vi "S8300E_COMPARE_LANMAC_SFCS_Auto.vi"() -> ()   [LabVIEW 2011]
panel:
  out "Expected MAC":string[](array[string])
  out "PORT1_MAC":string
  out "UUT MAC List":string
  out "CMD-LIST":cluster{string, string, string, string}[](array[cluster])
  out "log msg":string
  out "VISA resource name out":refnum<visa-resource-name>
  out "BEGIN TIME":u32
  out "進行狀況":string
  # "Error Code:MAC-PORT1\nError Code:MAC-PORT2\nError Code:MAC-PORT3"
  # "2014-12-12"
  # "S8300E UUT 3 Ports MAC (接UART COM9)"
  # "Step1:PQAW_MAC.LOG  contains MAC1 information\nStep2:Compare UUT MAC with PQAW_MAC.Log"
  # "Auto-Test\n自動測試"
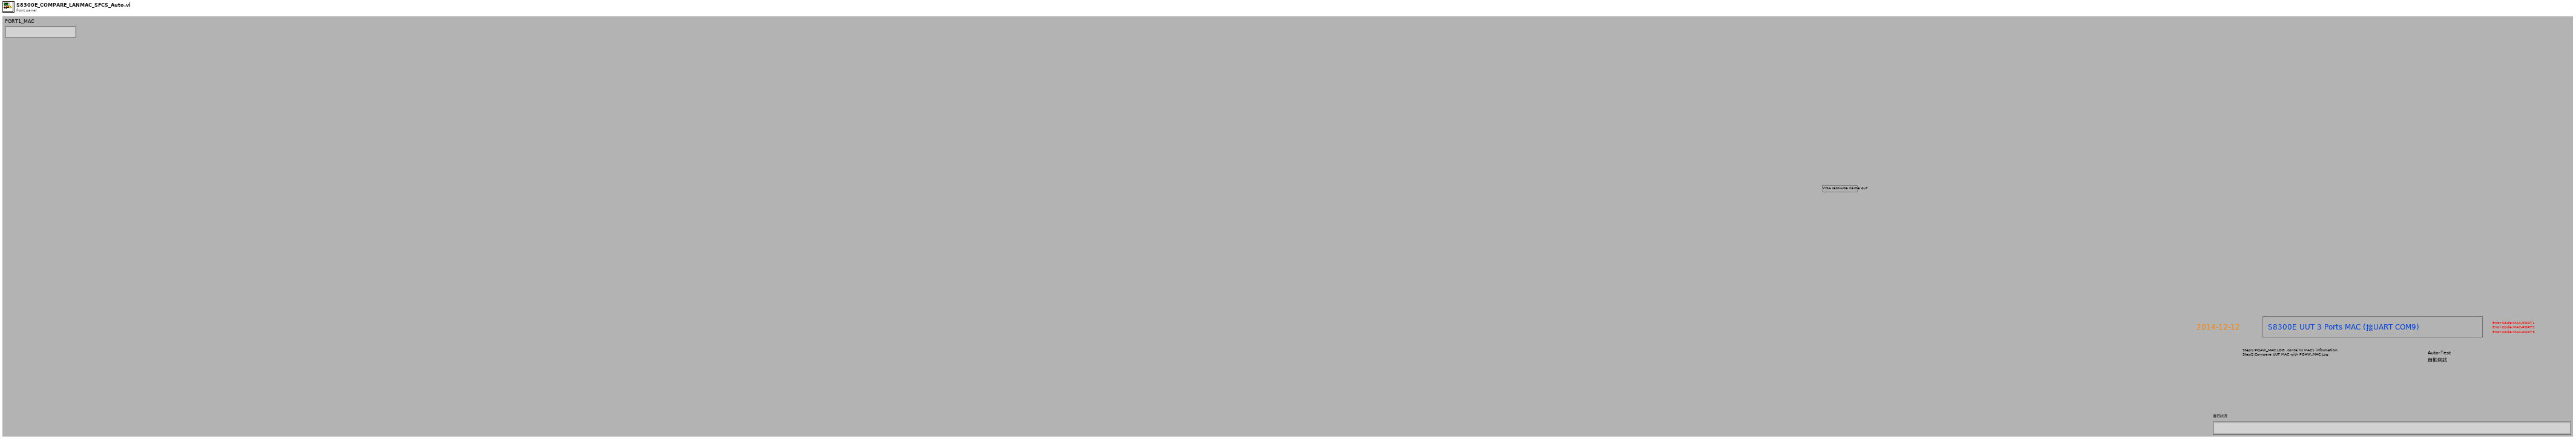
[diagram p1: front panel]
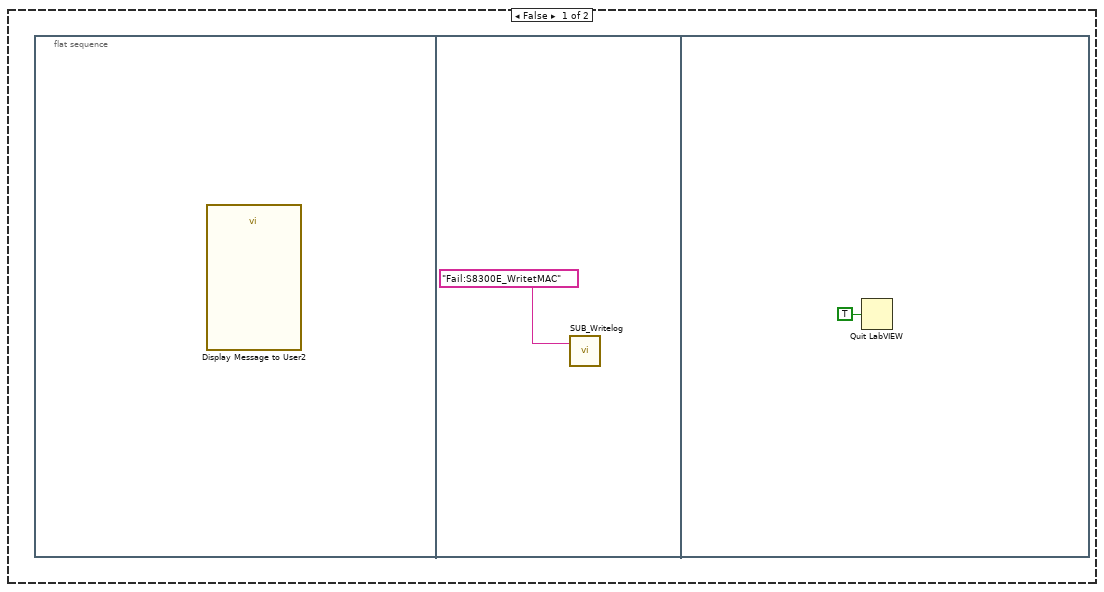
[diagram p3: hidden frame]
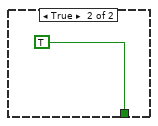
[diagram p9: hidden frame]
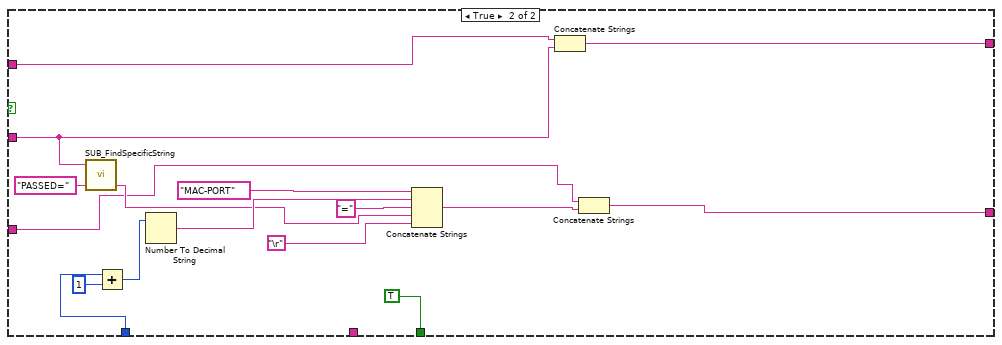
[diagram p11: hidden frame]
diagram:
  n1 = flat-sequence {
    frame #0 {
      n2 = Tick Count (ms)() -> (millisecond timer value=→"BEGIN TIME":u32)
    }
    frame #1 {
      n3 = property on="進行狀況" class="Str"("Blinking"=TRUE) -> ()  [unwired: 2 in, 2 out]
      "進行狀況" <- "進入測試準備中...." ("進行狀況")
      "PORT1_MAC" <- ""
    }
    frame #2 {
      n4 = call "SUB_SearchFile_inFolder.vi"("Search Filename in Folder"="S8300E_sfcs_misc.txt") -> ("File Existing True/Flase"=w5:bool)  [unwired: 1 in]
      n5 = case shown="False" w5 {
        frame False {
          n6 = flat-sequence {
            frame #0 {
              n7 = call "Display Message to User"() -> ()  [unwired: 10 in, 2 out]
            }
            frame #1 {
              n8 = call "SUB_Writelog.vi"("Pass/Fail"="Fail:S8300E_COMPARE_LANMAC_SFCS_Auto") -> ()  [unwired: 2 in]
            }
            frame #2 {
              n9 = Quit LabVIEW(quit? (T)=TRUE) -> ()
            }
          }
        }
        frame True {
        }
      }
    }
    frame #3 {
      n10 = call "SUB_SearchFile_inFolder.vi"("Search Filename in Folder"="PQAW_MAC.LOG") -> ("File Existing True/Flase"=w9:bool)  [unwired: 1 in]
      n11 = case shown="True" w9 {
        frame False {
          n12 = flat-sequence {
            frame #0 {
              n13 = call "Display Message to User2"() -> ()  [unwired: 10 in, 2 out]
            }
            frame #1 {
              n14 = call "SUB_Writelog.vi"("Pass/Fail"="Fail:S8300E_WritetMAC") -> ()  [unwired: 2 in]
            }
            frame #2 {
              n15 = Quit LabVIEW(quit? (T)=TRUE) -> ()
            }
          }
        }
        frame True {
          n16 = call "SUB_Read_specifFile.vi"("name or relative path"="PQAW_MAC.LOG" ("Search Filename in Folder")) -> ("text"=w20:string)  [unwired: 1 in, 1 out]
          n17 = call "SUB_FindSpecificString.vi"("Find this String"="LAN_MAC=", "String data"=w20) -> ("before \"; \" string"=w18:string, "Found"=w14:bool)  [unwired: 2 in]
          n18 = local write "PORT1_MAC"(w18) -> ()
          n19 = String Length(string=w18) -> (length=w17:i32)
          n20 = Equal?(x=w17, y=12) -> (x = y?=w13:bool)
          n21 = And(x=w14, y=w13) -> (x .and. y?=w15:bool)
          n22 = case shown="False" w15 {
            frame False {
              n23 = flat-sequence {
                frame #0 {
                  n24 = call "Display Message to User3"() -> ()  [unwired: 10 in, 2 out]
                }
                frame #1 {
                  n25 = call "SUB_Writelog.vi"("Pass/Fail"="Fail:S8300E_COMPARE_LANMAC_SFCS_Auto") -> ()  [unwired: 2 in]
                }
                frame #2 {
                  n26 = Quit LabVIEW(quit? (T)=TRUE) -> ()
                }
              }
            }
            frame True {
            }
          }
        }
      }
    }
    frame #4 {
      n27 = local read "PORT1_MAC"() -> (w34:string)
      n28 = call "SUB_Gen3ports_MACString.vi"("Port1-MAC Input"=w34) -> ("port3-MAC"=w25:string, "port2-MAC"=w26:string, "port1-MAC"=w27:string)  [unwired: 2 in]
      n29 = Concatenate Strings("./mac.sh -r -e  1", "\r") -> (w51:string)
      n30 = Concatenate Strings("PASSED=", w27) -> (w32:string)
      n31 = Concatenate Strings("PASSED=", w26) -> (w30:string)
      n32 = Concatenate Strings("./mac.sh -r -e  2", "\r") -> (w47:string)
      n33 = Concatenate Strings("PASSED=", w25) -> (w28:string)
      n34 = Concatenate Strings("./mac.sh -r -e  3", "\r") -> (w43:string)
      n35 = Bundle(w51, w32, "Checking MAC-PORT1..", "MAC-PORT1") -> (w38:cluster{string, string, string, string})  [unwired: 1 in]
      n36 = Bundle(w47, w30, "Checking MAC-PORT2...", "MAC-PORT2") -> (w37:cluster{string, string, string, string})  [unwired: 1 in]
      n37 = Build Array(w27, w26, w25) -> (→"Expected MAC":string[])
      n38 = Bundle(w43, w28, "Checking MAC-PORT3...", "MAC-PORT3") -> (w36:cluster{string, string, string, string})  [unwired: 1 in]
      n39 = Build Array(w38, w37, w36) -> (→"CMD-LIST":cluster{string, string, string, string}[])
    }
    frame #5 {
      n40 = case shown="True" TRUE {
        frame False {
        }
        frame True {
          n41 = call "SUB_COM1_CLOSE.vi"("VISA resource name"=refnum<visa-resource-name> "COM9") -> ()  [unwired: 3 in]
        }
      }
    }
    frame #6 {
      n42 = case shown="True" TRUE {
        frame False {
        }
        frame True {
          w58 = "\r"
          n43 = call "SUB_COM9_INIT.vi"("baud rate"=u32 115200) -> ("VISA resource name out"=w62:refnum<visa-resource-name>)  [unwired: 1 in, 1 out]
          "VISA resource name out" <- w62
          n44 = Concatenate Strings(w58, w58, w58) -> (w57:string)
          n45 = call "SUB_COM1Wrt.vi"("VISA resource name"=w62, "write buffer"=w57) -> ("duplicate VISA resource name"=w59:refnum<visa-resource-name>)  [unwired: 1 in, 1 out]
          n46 = call "SUB_ContinueCom1Read.vi"("Numeric"=1200, "duplicate VISA resource name 2"=w59) -> ()  [unwired: 1 in, 3 out]
        }
      }
    }
    frame #7 {
      n47 = case shown="True" TRUE {
        frame False {
        }
        frame True {
          n48 = while {
            stop <- w73 stop-if-true
            w64 = "\r"
            n49 = local read "VISA resource name out"() -> (w66:refnum<visa-resource-name>)
            n50 = Tick Count (ms)() -> (millisecond timer value=w71:u32)
            n51 = Concatenate Strings(w64, w64, w64) -> (w65:string)
            n52 = call "SUB_COM1Wrt.vi"("VISA resource name"=w66, "write buffer"=w65) -> ("duplicate VISA resource name"=w72:refnum<visa-resource-name>)  [unwired: 1 in, 1 out]
            n53 = call "SUB_READ_COM1_FindString_timeout.vi"("Find this String"="s8300e_func_test#", "Timeout Seccond"=2.0, "Begin time"=w71, "duplicate VISA resource name 2"=w72) -> ("Output String"=w67:string, "Found String"=w68:bool)  [unwired: 1 in, 1 out]
            n54 = case shown="False" w68 {
              tunnel: [w75 TRUE] -> w73
              tunnel: w67 -> [w74 _]
              frame False {
                n55 = call "SUB_YESNO.vi"("Debug View"=w74, "Status"="UART無正確反應!需有S8300E字串") -> ("yes/no"=w78:enum32{"No Selection", "Yes", "No", "None"})  [unwired: 1 in]
                n56 = Equal?(x=w78, y=enum32{"No Selection", "Yes", "No", "None"}."No") -> (x = y?=w76:bool)
                n57 = case shown="True" w76 {
                  tunnel: [_ w80] -> w75
                  frame False {
                  }
                  frame True {
                    n58 = flat-sequence {
                      tunnel: [w84] -> w80
                      frame #0 {
                        n59 = call "SUB_Writelog.vi"("Pass/Fail"="Fail:S8300E_COMPARE_LANMAC_SFCS_Auto") -> ()  [unwired: 2 in]
                      }
                      frame #1 {
                        n60 = call "SUB_SFCS_SendResult.vi"("ErrorCode"="UART", "PASS_Fail (1/0)"=i8 0) -> ()  [unwired: 1 out]
                      }
                      frame #2 {
                        w84 = TRUE ("quit? (T)")
                        n61 = Quit LabVIEW(quit? (T)=w84) -> ()
                      }
                    }
                  }
                }
              }
              frame True {
              }
            }
          }
        }
      }
    }
    frame #8 {
      n62 = local read "CMD-LIST"() -> (w88:cluster{string, string, string, string}[])
      n63 = Array Size(array=w88) -> (size(s)=w91:i32)
      n64 = for {
        N: w91 -> [_]
        shift-right: [w96] -> w89
        shift-left: "" -> [w95]
        shift-right: [w93] -> w86
        shift-left: "" -> [w92]
        i -> [w94]
        n65 = while {
          tunnel: w94 -> [w115]
          tunnel: [w107] -> w96
          tunnel: w95 -> [w106]
          tunnel: w94 -> [w99]
          tunnel: [w98] -> w93
          tunnel: w92 -> [w97]
          stop <- w109 stop-if-true
          n66 = local read "VISA resource name out"() -> (w111:refnum<visa-resource-name>)
          n67 = local read "CMD-LIST"() -> (w105:cluster{string, string, string, string}[])
          n68 = Index Array(array=w105, index=w115) -> (element=w104:cluster{string, string, string, string})
          n69 = Unbundle(w104) -> (w103:string, w101:string, w102:string, w100:string)
          n70 = call "SUB_COM1Wrt.vi"("VISA resource name"=w111, "write buffer"=w103) -> ("duplicate VISA resource name"=w114:refnum<visa-resource-name>)  [unwired: 1 in, 1 out]
          n71 = Tick Count (ms)() -> (millisecond timer value=w113:u32)
          n72 = call "SUB_READ_COM1_FindString_timeout.vi"("Find this String"=w101, "Timeout Seccond"=2.0, "Begin time"=w113, "duplicate VISA resource name 2"=w114) -> ("Output String"=w108:string, "Found String"=w110:bool)  [unwired: 1 in, 1 out]
          n73 = local write "進行狀況"(w102) -> ()
          n74 = case shown="False" w110 {
            tunnel: [_ TRUE] -> w109
            tunnel: w108 -> [w117 w151]
            tunnel: [w131 w156] -> w107
            tunnel: w106 -> [w131 w155]
            tunnel: w100 -> [w130 _]
            tunnel: w99 -> [w124 w147]
            tunnel: [w126 w143] -> w98
            tunnel: w97 -> [w126 w142]
            frame False {
              n75 = local read "Expected MAC"() -> (w125:string[])
              n76 = local read "進行狀況"() -> (w128:string)
              n77 = Concatenate Strings("如下系統回傳值" ("string"), "\r", w117) -> (w116:string)
              n78 = Index Array(array=w125, index=w124) -> (element=w122:string)
              n79 = Concatenate Strings("期望MAC 值=" ("string"), w122, "\r") -> (w120:string)
              n80 = Concatenate Strings(w120, "\r", w128) -> (w127:string)
              n81 = call "SUB_YESNO.vi"("Debug View"=w116, "Status"=w127) -> ("yes/no"=w134:enum32{"No Selection", "Yes", "No", "None"})  [unwired: 1 in]
              n82 = Equal?(x=w134, y=enum32{"No Selection", "Yes", "No", "None"}."No") -> (x = y?=w132:bool)
              n83 = case shown="True" w132 {
                tunnel: w130 -> [_ w135]
                frame False {
                }
                frame True {
                  n84 = flat-sequence {
                    tunnel: [w137] -> w136
                    tunnel: w135 -> [w137]
                    tunnel: w136 -> [w139]
                    frame #0 {
                      n85 = call "SUB_Writelog.vi"("Pass/Fail"="Fail:S8300E_COMPARE_LANMAC_SFCS_Auto") -> ()  [unwired: 2 in]
                    }
                    frame #1 {
                      n86 = call "SUB_SFCS_SendResult.vi"("ErrorCode"=w139, "PASS_Fail (1/0)"=i8 0) -> ()  [unwired: 1 out]
                    }
                    frame #2 {
                      n87 = Quit LabVIEW(quit? (T)=TRUE) -> ()
                    }
                  }
                }
              }
            }
            frame True {
              n88 = call "SUB_FindSpecificString.vi"("Find this String"="PASSED=", "String data"=w151) -> ("before \"; \" string"=w149:string)  [unwired: 2 in, 1 out]
              n89 = Add(x=w147, y=1) -> (x+y=w145:i32)
              n90 = Number To Decimal String(number=w145) -> (decimal integer string=w153:string)  [unwired: 1 in]
              n91 = Concatenate Strings("MAC-PORT" ("string"), w153, "=" ("string"), w149, "\r") -> (w144:string)
              n92 = Concatenate Strings(w155, w151) -> (w156:string)
              n93 = Concatenate Strings(w142, w144) -> (w143:string)
            }
          }
        }
      }
      "log msg" <- w89
      "UUT MAC List" <- w86
    }
    frame #9 {
      n94 = call "SUB_COM1_CLOSE.vi"("VISA resource name"=refnum<visa-resource-name> "COM9") -> ()  [unwired: 3 in]
    }
    frame #10 {
      n95 = local read "log msg"() -> (w159:string)
      n96 = local read "BEGIN TIME"() -> (w165:u32)
      n97 = Tick Count (ms)() -> (millisecond timer value=w164:u32)
      n98 = call "SUB_CAL_TESTTIME.vi"("Test Item name"="S8300E_COMPARE_LANMAC_SFCS_Auto", "Stop tick time"=w164, "Start tick time"=w165) -> ("Test Time output"=w161:string)  [unwired: 2 in]
      n99 = Concatenate Strings("Pass:S8300E_COMPARE_LANMAC_SFCS_Auto", "\n", w159, w161) -> (w162:string)
      n100 = call "SUB_Writelog.vi"("Pass/Fail"=w162) -> ()  [unwired: 2 in]
    }
    frame #11 {
      n101 = Request Deallocation(TRUE ("flag")) -> ()
    }
    frame #12 {
      n102 = Quit LabVIEW(quit? (T)=TRUE ("stop? (T)")) -> ()
    }
  }
